vi "LINX - Photocell.vi"() -> ()   [LabVIEW 2011, in "LVH-LINX.lvlib"]
doc: "Measure light intensity using a photocell."
uses:
  vi.lib/LabVIEW Hacker/LINX/LVH-LINX.lvlib
panel:
  out "Photocell Value":u8(slide) scale=0.0..100.0
  in  "AI Channel":u8
  in  "Serial Port":refnum<visa-resource-name>
  out "Loop Rate (Hz)":u32
  in  "Stop Button":bool
  # "Circuit Schematic"
  # "LINX Device Settings"
  # "Photocell Value"
  # "Photocell Example (Serial Interface)\n\nThis example demonstrates how to measure light intensity using a photocell.\n\nInstructions\n1. Select the COM Port associated with the LINX Device.\n2. Select the Analog Channel connected to the photocell.\n3. Click the Run Arrow."
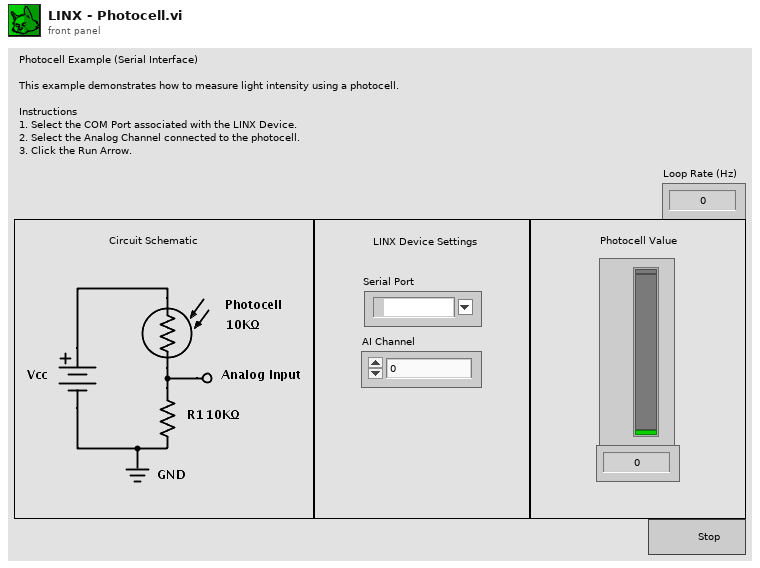
[diagram p1: front panel]
types:
  T1 = typedef "LVH-LINX.lvlib/LINX Ref.ctl" = cluster{"Platform":T2, "Interface":T3, "LINX Device Config":T4}
  T2 = typedef "LVH-LINX.lvlib/Platform.ctl" = enum16{"LINX", "myRIO"}
  T3 = typedef "LVH-LINX.lvlib/Interface.ctl" = enum16{"Serial", "TCP"}
  T4 = typedef "LVH-LINX.lvlib/Device.lvlib/LINX Device Config.ctl" = cluster{"Interface":T3, "COM Port":refnum<visa-resource-name>, "TCP Configuration":T5, "Device Family":T6, "Device ID":u8, "Device Name":string, "TCP Ref":refnum<k5>}
  T5 = typedef "LVH-LINX.lvlib/Device.lvlib/TCP Config.ctl" = cluster{"IP Address":string, "Port":u16}
  T6 = typedef "LVH-LINX.lvlib/Device Family.ctl" = enum8{"National Instruments", "Digilent", "Arduino"}
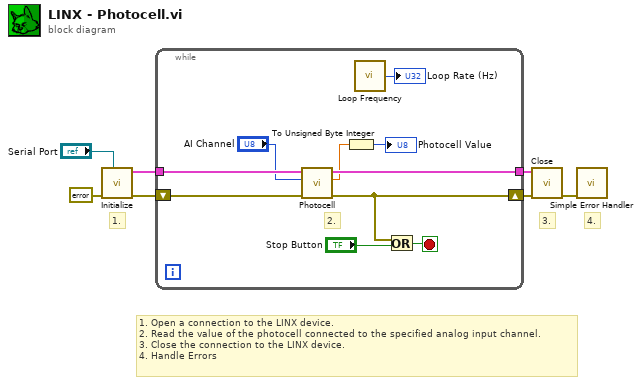
[diagram p0: block diagram]
diagram:
  # "1. Open a connection to the LINX device.\n2. Read the value of the photocell connected to the specified analog input channel.\n3. Close the connection to the LINX device.\n4. Handle Errors"
  # "4."
  # "3."
  # "1."
  n1 = call "Initialize.vi"("Serial Port"="Serial Port", "Error In"=errorcluster {"status"=FALSE, "code"=0, "source"=""}) -> ("Error Out"=w6:errorcluster, "LINX Ref"=w7:T1)  [unwired: 7 in, 1 out]
  n2 = while {
    tunnel: w7 -> [w14]
    tunnel: [w13] -> w5
    shift-right: [w12] -> w4
    shift-left: w6 -> [w11]
    stop <- w17 stop-if-true
    # "2."
    n3 = call "Photocell.vi"("Error In"=w11, "AI Channel"="AI Channel", "LINX Resource"=w14) -> ("Error Out"=w12:errorcluster, "Value (0-100)"=w8:dbl, "LINX Resource"=w13:T1)  [unwired: 6 in]
    n4 = To Unsigned Byte Integer(number=w8) -> (unsigned 8bit integer=→"Photocell Value":u8)
    n5 = call "Loop Frequency.vi"() -> ("Loop Rate (Hz)"=→"Loop Rate (Hz)":u32)
    n6 = Or(x=w12, y="Stop Button") -> (x .or. y?=w17:bool)
  }
  n7 = call "Close.vi"("Error In"=w4, "LINX Resource"=w5) -> ("Error Out"=w2:errorcluster)  [unwired: 8 in, 1 out]
  n8 = call <vilib>:"Simple Error Handler.vi"("error in (no error)"=w2) -> ()  [unwired: 4 in, 5 out]
